vi "SubSystems.vi"(8 "error in":errorcluster) -> ()   [LabVIEW 2015]
doc: "This VI calls the various robot subsystems that will then run in parallel. New subSystems will automatlically script code to make the call."
uses:
  <vilib>/Rock Robotics/WPI/Camera/WPI_CameraImageSize.ctl
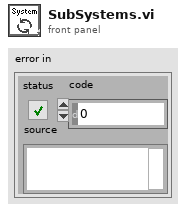
[diagram p1: front panel]
types:
  T1 = typedef "WPI_CameraImageSize.ctl" = enum16{"640x480", "320x240", "160x120", "Custom"}
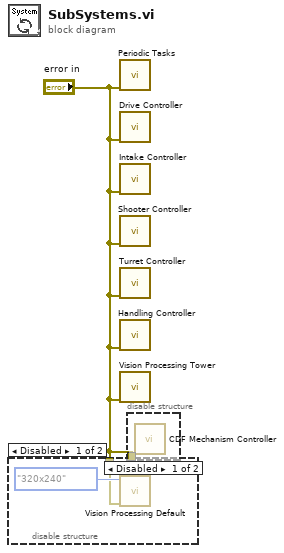
[diagram p0: block diagram]
diagram:
  n1 = disable-structure shown="Disabled" {
    disable-tunnel: "error in" -> [w2 _]
    frame Disabled {
      n2 = call "Vision Processing Default.vi"("error in (no error)"=w2, "Image Size"=WPI_CameraImageSize."320x240") -> ()  [unwired: 6 in]
    }
    frame Enabled {
    }
  }
  n3 = call "Periodic Tasks.vi"("error in"="error in") -> ()  [unwired: 1 in, 10 out]
  n4 = call "Drive Controller.vi"("error in"="error in") -> ()  [unwired: 11 in]
  n5 = call "Intake Controller.vi"("error in"="error in") -> ()  [unwired: 11 in]
  n6 = call "Shooter Controller.vi"("error in"="error in") -> ()  [unwired: 11 in]
  n7 = call "Turret Controller.vi"("error in"="error in") -> ()  [unwired: 11 in]
  n8 = call "Handling Controller.vi"("error in"="error in") -> ()  [unwired: 11 in]
  n9 = call "Vision Processing Tower.vi"("error in (no error)"="error in") -> ()  [unwired: 7 in]
  n10 = disable-structure shown="Disabled" {
    disable-tunnel: "error in" -> [w4 _]
    frame Disabled {
      n11 = call "CDF Mechanism Controller.vi"("error in"=w4) -> ()  [unwired: 11 in]
    }
    frame Enabled {
    }
  }
